vi "Main.vi"() -> ()   [LabVIEW 2015]
doc: "This template is for the Queued Message Handler design pattern.\n\nThe Event Handling Loop generates messages based on user interface actions.\n\nThe Message Handling Loop processes messages generated by the Event Handling Loop, or by other messages. The messages are string values, so new messages can be added easily to the Message Cases case structure in the Message Handling Loop. Each message cluster can also provide an optional value for Message Data, which is a variant that can be converted to whatever message-specific data is required."
uses:
  controls/UI Data.ctl
  support/Boiler System Globals.vi
  support/Message Queue/Message Queue.lvlib
  support/User Event - Stop/User Event - Stop.lvlib
  Boiler/Boiler.lvlib
panel:
  out "Display <Replace Me>":string
  in  "Do Something Else <Replace Me>":bool
  in  "Do Something <Replace Me>":bool
  in  "Stop Button":bool
  # "These controls have associated \"Value Changed\" events configured in the Event Structure on the diagram.\n\nReplace them (and reconfigure the Event Structure) with the controls you need for your application."
  # "This template is for the Queued Message Handler design pattern.\n\nSee the block diagram for more information on how to use this template."
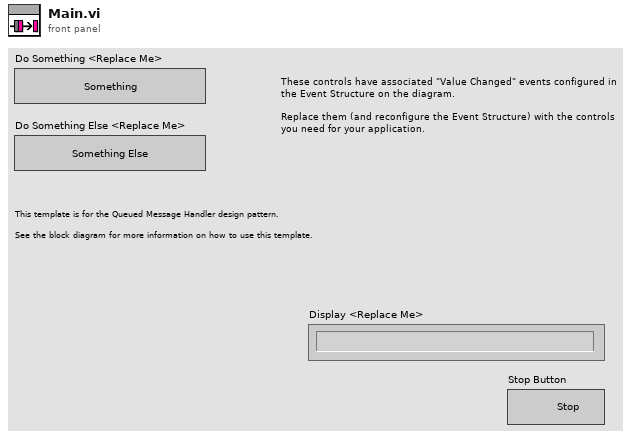
[diagram p1: front panel]
types:
  T1 = typedef "UI Data.ctl" = cluster{"Boolean <Replace Me>":bool, "String <Replace Me>":string, "Numeric <Replace Me>":dbl, "Do Something Ref":refnum<vi>, "Do Something Else Ref":refnum<vi>, "Data Display Ref":refnum<vi>, "Stop Button Ref":refnum<vi>}
  T2 = typedef "Notifiers.ctl" = cluster{"Handshake":refnum<notifier>, "Flame Level":refnum<notifier>, "Controller Exit":refnum<notifier>, "Boiler Exit":refnum<notifier>}
  T3 = typedef "Message Queue.lvlib/All Message Queues.ctl" = cluster{"MHL":refnum<queue>, "Boiler Controller":refnum<queue>, "Boiler":refnum<queue>}
  T4 = enum32{"invalid app kind", "Development System", "Run Time System", "Student Edition", "Embedded LabVIEW", "Evaluation", "Custom"}
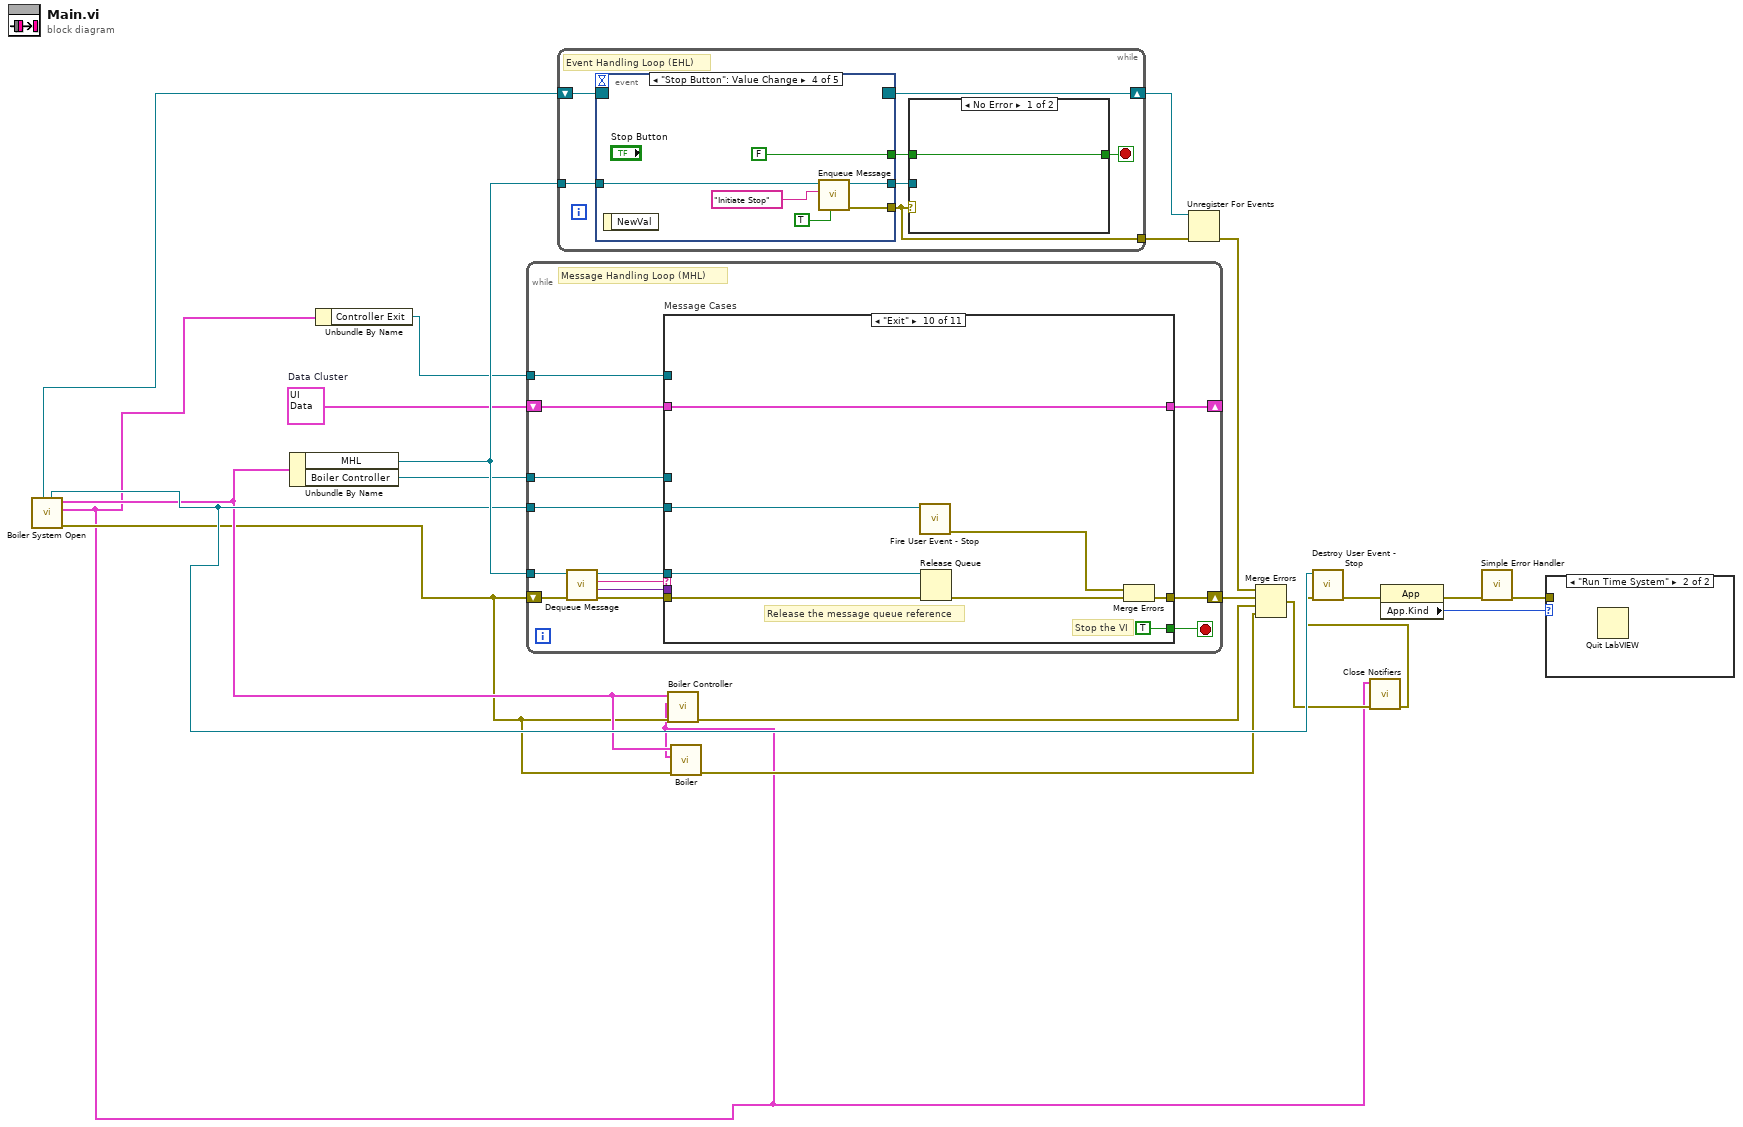
[diagram p0: block diagram]
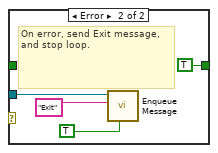
[diagram p3: hidden frame]
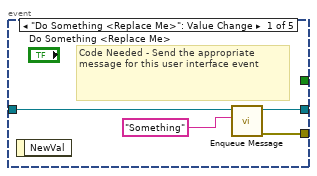
[diagram p4: hidden frame]
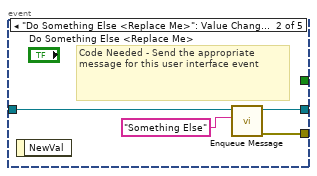
[diagram p5: hidden frame]
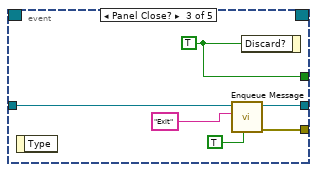
[diagram p6: hidden frame]
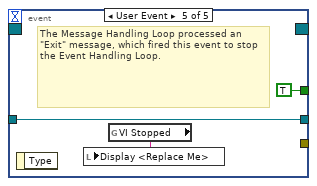
[diagram p7: hidden frame]
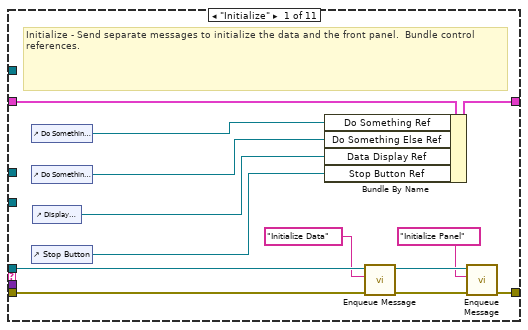
[diagram p8: hidden frame]
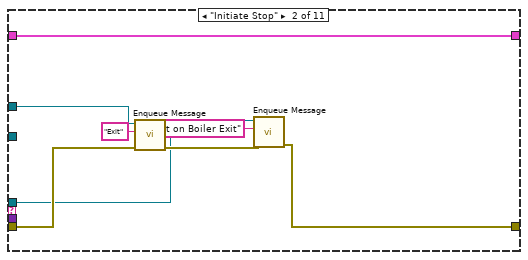
[diagram p9: hidden frame]
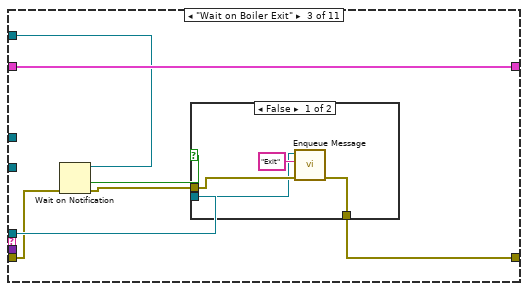
[diagram p10: hidden frame]
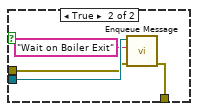
[diagram p11: hidden frame]
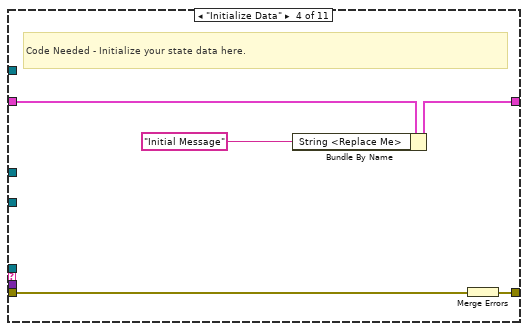
[diagram p12: hidden frame]
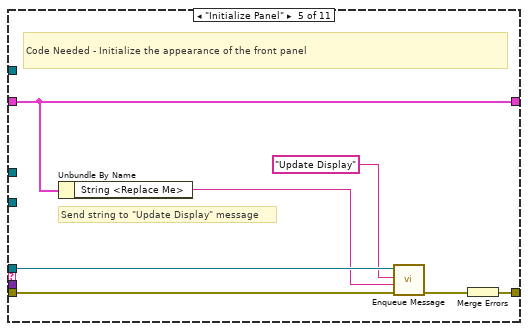
[diagram p13: hidden frame]
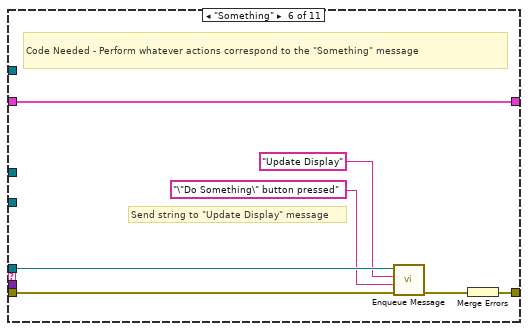
[diagram p14: hidden frame]
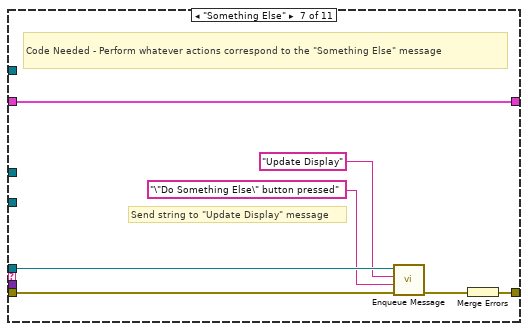
[diagram p15: hidden frame]
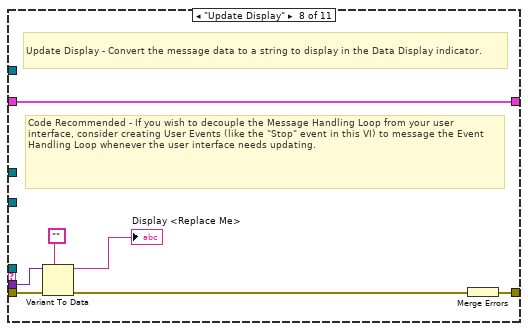
[diagram p16: hidden frame]
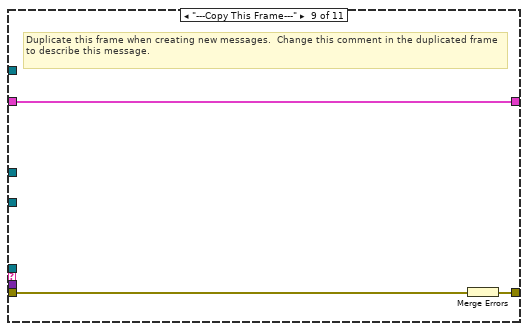
[diagram p17: hidden frame]
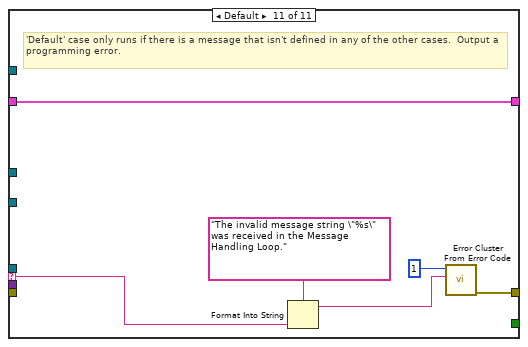
[diagram p18: hidden frame]
diagram:
  w15 = T1 {"Boolean <Replace Me>"=TRUE, "String <Replace Me>"="", "Numeric <Replace Me>"=0.0, "Do Something Ref"=refnum, "Do Something Else Ref"=refnum, "Data Display Ref"=refnum, "Stop Button Ref"=refnum}  # Data Cluster
  n1 = call "Boiler System Open.vi"() -> ("error out"=w6:errorcluster, "Notifiers"=w1:T2, "Message Queues"=w7:T3, "User Event - Stop"=w8:refnum<user-event>, "Stop Event Registration Refnum"=w9:refnum<event-registration>)  [unwired: 7 in]
  n2 = Unbundle By Name(w7) -> ("MHL"=w20:refnum<queue>, "Boiler Controller"=w13:refnum<queue>)
  n3 = Unbundle By Name(w1) -> ("Controller Exit"=w4:refnum<notifier>)
  n4 = while {
    tunnel: w20 -> [w24]
    shift-right: [w33] -> _
    shift-left: w15 -> [w34]
    tunnel: w8 -> [w30]
    shift-right: [w31] -> w21
    shift-left: w6 -> [w29]
    tunnel: w13 -> [w23]
    tunnel: w4 -> [w22]
    stop <- w32 stop-if-true
    # "Message Handling Loop (MHL)"
    n5 = call "Dequeue Message.vi"("error in (no error)"=w29, "Message Queue"=w24) -> ("error out"=w28:errorcluster, "Message Data"=w26:variant, "Message"=w27:string, "dup Message Queue"=w25:refnum<queue>)  [unwired: 6 in]
    n6 = case "Message Cases" shown="\"Exit\"" w27 {
      selector: w27 -> [_ _ _ _ _ _ _ _ _ _ w118]
      tunnel: w25 -> [w43 w49 w59 _ w79 w85 w92 _ _ w114 _]
      tunnel: w28 -> [w46 w51 w58 w75 w80 w87 w94 w101 w106 w107 _]
      tunnel: [w47 w50 w56 w71 w81 w88 w95 w102 w104 w110 w116] -> w31
      tunnel: w34 -> [w40 w55 w62 w74 w82 w89 w96 w103 w105 w113 w120]
      tunnel: [w39 w55 w62 w73 w82 w89 w96 w103 w105 w113 w120] -> w33
      tunnel: [_ _ _ _ _ _ _ _ _ TRUE _] -> w32
      tunnel: w26 -> [_ _ _ _ _ _ _ w100 _ _ _]
      tunnel: w30 -> [_ _ _ _ _ _ _ _ _ w109 _]
      tunnel: w23 -> [_ w54 _ _ _ _ _ _ _ _ _]
      tunnel: w22 -> [_ _ w61 _ _ _ _ _ _ _ _]
      frame "Initialize" {
        # "Initialize - Send separate messages to initialize the data and the front panel.  Bundle control references."
        n7 = control-ref of="Do Something <Replace Me>"() -> (w38:refnum<vi>)
        n8 = control-ref of="Do Something Else <Replace Me>"() -> (w37:refnum<vi>)
        n9 = control-ref of="Stop Button"() -> (w35:refnum<vi>)
        n10 = control-ref of="Display <Replace Me>"() -> (w36:refnum<vi>)
        n11 = Bundle By Name(cluster=w40, "Do Something Ref"=w38, "Do Something Else Ref"=w37, "Data Display Ref"=w36, "Stop Button Ref"=w35) -> (w39:T1)
        n12 = call "Enqueue Message.vi"("error in (no error)"=w46, "Message"="Initialize Data", "Message Queue"=w43) -> ("error out"=w45:errorcluster, "dup Message Queue"=w44:refnum<queue>)  [unwired: 7 in]
        n13 = call "Enqueue Message.vi"("error in (no error)"=w45, "Message"="Initialize Panel", "Message Queue"=w44) -> ("error out"=w47:errorcluster)  [unwired: 7 in, 1 out]
      }
      frame "Initiate Stop" {
        n14 = call "Enqueue Message.vi"("error in (no error)"=w51, "Message"="Exit", "Message Queue"=w54) -> ("error out"=w52:errorcluster)  [unwired: 7 in, 1 out]
        n15 = call "Enqueue Message.vi"("error in (no error)"=w52, "Message"="Wait on Boiler Exit", "Message Queue"=w49) -> ("error out"=w50:errorcluster)  [unwired: 7 in, 1 out]
      }
      frame "Wait on Boiler Exit" {
        n16 = Wait on Notification(notifier=w61, error in (no error)=w58) -> (timed out?=w60:bool, error out=w57:errorcluster)  [unwired: 2 in, 2 out]
        n17 = case shown="False" w60 {
          tunnel: w59 -> [w63 w70]
          tunnel: w57 -> [w65 w68]
          tunnel: [w64 w67] -> w56
          frame False {
            n18 = call "Enqueue Message.vi"("error in (no error)"=w65, "Message"="Exit", "Message Queue"=w63) -> ("error out"=w64:errorcluster)  [unwired: 7 in, 1 out]
          }
          frame True {
            n19 = call "Enqueue Message.vi"("error in (no error)"=w68, "Message"="Wait on Boiler Exit", "Message Queue"=w70) -> ("error out"=w67:errorcluster)  [unwired: 7 in, 1 out]
          }
        }
      }
      frame "Initialize Data" {
        # "Code Needed - Initialize your state data here."
        n20 = Bundle By Name(cluster=w74, "String <Replace Me>"="Initial Message" ("Initial Message")) -> (w73:T1)
        n21 = Merge Errors(w75) -> (w71:errorcluster)
      }
      frame "Initialize Panel" {
        # "Send string to \"Update Display\" message"
        # "Code Needed - Initialize the appearance of the front panel"
        n22 = Unbundle By Name(w82) -> ("String <Replace Me>"=w76:string)
        n23 = call "Enqueue Message.vi"("error in (no error)"=w80, "Message Data"=w76, "Message"="Update Display", "Message Queue"=w79) -> ("error out"=w78:errorcluster)  [unwired: 6 in, 1 out]
        n24 = Merge Errors(w78) -> (w81:errorcluster)
      }
      frame "Something" {
        # "Send string to \"Update Display\" message"
        # "Code Needed - Perform whatever actions correspond to the \"Something\" message"
        n25 = call "Enqueue Message.vi"("error in (no error)"=w87, "Message Data"="\"Do Something\" button pressed" ("\"Do Something\" button pressed"), "Message"="Update Display", "Message Queue"=w85) -> ("error out"=w86:errorcluster)  [unwired: 6 in, 1 out]
        n26 = Merge Errors(w86) -> (w88:errorcluster)
      }
      frame "Something Else" {
        # "Send string to \"Update Display\" message"
        # "Code Needed - Perform whatever actions correspond to the \"Something Else\" message"
        n27 = call "Enqueue Message.vi"("error in (no error)"=w94, "Message Data"="\"Do Something Else\" button pressed" ("\"Do Something Else\" button pressed"), "Message"="Update Display", "Message Queue"=w92) -> ("error out"=w93:errorcluster)  [unwired: 6 in, 1 out]
        n28 = Merge Errors(w93) -> (w95:errorcluster)
      }
      frame "Update Display" {
        # "Code Recommended - If you wish to decouple the Message Handling Loop from your user interface, consider creating User Events (like the \"Stop\" event in this VI) to message the Event Handling Loop whenever the user interface needs updating."
        # "Update Display - Convert the message data to a string to display in the Data Display indicator."
        n29 = Variant To Data(error in=w101, type="", Variant=w100) -> (data=→"Display <Replace Me>":string, error out=w98:errorcluster)
        n30 = Merge Errors(w98) -> (w102:errorcluster)
      }
      frame "---Copy This Frame---" {
        # "Duplicate this frame when creating new messages.  Change this comment in the duplicated frame to describe this message."
        n31 = Merge Errors(w106) -> (w104:errorcluster)
      }
      frame "Exit" {
        # "Stop the VI"
        # "Release the message queue reference"
        n32 = call "Fire User Event - Stop.vi"("User Event - Stop"=w109) -> ("error out"=w108:errorcluster)  [unwired: 10 in]
        n33 = Release Queue(queue=w114, error in (no error)=w107) -> (error out=w111:errorcluster)  [unwired: 1 in, 2 out]
        n34 = Merge Errors(w108, w111) -> (w110:errorcluster)
      }
      frame Default {
        # "'Default' case only runs if there is a message that isn't defined in any of the other cases.  Output a programming error."
        n35 = Format Into String(format string="The invalid message string \"%s\" was received in the Message Handling Loop." ("Unknown Message Error Text"), w118) -> (resulting string=w115:string)  [unwired: 2 in, 1 out]
        n36 = call <vilib>:"Error Cluster From Error Code.vi"("error message (\"\")"=w115, "error code (0)"=1) -> ("error out"=w116:errorcluster)  [unwired: 7 in]
      }
    }
  }
  n37 = while {
    tunnel: w20 -> [w127]
    tunnel: [w123] -> w17
    shift-right: [w121] -> w16
    shift-left: w9 -> [w122]
    stop <- w125 stop-if-true
    # "Event Handling Loop (EHL)"
    n38 = event shown="[3] \"Stop Button\": Value Change" {
      selector: w122 -> [_ _ _ _ _]
      dyn-events: [_ _ _ _ _] -> w121
      timeout: _ -> [_ _ _ _ _]
      tunnel: [_ _ w146 FALSE ("Discard?") TRUE ("Discard?")] -> w126
      tunnel: w127 -> [w136 w140 w145 w152 w155]
      tunnel: [w135 w138 w144 w151 _] -> w123
      tunnel: [w134 w139 w143 w149 w155] -> w124
      event "Do Something <Replace Me>": Value Change {
        # "Code Needed - Send the appropriate message for this user interface event"
        n39 = event-data() -> ()  [unwired: 1 in, 1 out]
        n40 = call "Enqueue Message.vi"("Message"="Something", "Message Queue"=w136) -> ("error out"=w135:errorcluster, "dup Message Queue"=w134:refnum<queue>)  [unwired: 8 in]
      }
      event "Do Something Else <Replace Me>": Value Change {
        # "Code Needed - Send the appropriate message for this user interface event"
        n41 = event-data() -> ()  [unwired: 1 in, 1 out]
        n42 = call "Enqueue Message.vi"("Message"="Something Else", "Message Queue"=w140) -> ("error out"=w138:errorcluster, "dup Message Queue"=w139:refnum<queue>)  [unwired: 8 in]
      }
      event Panel Close? {
        w146 = TRUE ("Discard?")
        n43 = event-data() -> ()  [unwired: 1 in, 1 out]
        n44 = call "Enqueue Message.vi"("Priority Message? (F)"=TRUE, "Message"="Exit", "Message Queue"=w145) -> ("error out"=w144:errorcluster, "dup Message Queue"=w143:refnum<queue>)  [unwired: 7 in]
        n45 = event-data("Discard?"=w146) -> ()  [unwired: 1 in, 1 out]
      }
      event "Stop Button": Value Change {
        n46 = event-data() -> ()  [unwired: 1 in, 1 out]
        n47 = call "Enqueue Message.vi"("Priority Message? (F)"=TRUE, "Message"="Initiate Stop", "Message Queue"=w152) -> ("error out"=w151:errorcluster, "dup Message Queue"=w149:refnum<queue>)  [unwired: 7 in]
      }
      event User Event {
        # "The Message Handling Loop processed an \"Exit\" message, which fired this event to stop the Event Handling Loop."
        n48 = event-data() -> ()  [unwired: 1 in, 1 out]
        n49 = global read "Boiler System Globals.vi" "VI Stopped"() -> (w153:string)
        n50 = local write "Display <Replace Me>"(w153) -> ()
      }
    }
    n51 = case shown="No Error" w123 {
      tunnel: [w128 TRUE ("Discard?")] -> w125
      tunnel: w126 -> [w128 _]
      tunnel: w124 -> [_ w131]
      frame No Error {
      }
      frame Error {
        # "On error, send Exit message, and stop loop."
        n52 = call "Enqueue Message.vi"("Priority Message? (F)"=TRUE, "Message"="Exit", "Message Queue"=w131) -> ()  [unwired: 7 in, 2 out]
      }
    }
  }
  n53 = call "Boiler Controller.vi"("error in"=w6, "Notifiers"=w1, "Message Queues"=w7) -> ("error out"=w14:errorcluster)  [unwired: 8 in]
  n54 = call "Boiler.vi"("error in"=w6, "Notifiers"=w1, "Message Queues"=w7) -> ("error out"=w5:errorcluster)  [unwired: 8 in]
  n55 = Unregister For Events(event registration refnum=w16, error in=w17) -> (error out=w18:errorcluster)
  n56 = Merge Errors(w18, w21, w14, w5) -> (w3:errorcluster)
  n57 = call "Close Notifiers.vi"("error in (no error)"=w3, "Cluster"=w1) -> ("error out"=w2:errorcluster)  [unwired: 9 in]
  n58 = call "Destroy User Event - Stop.vi"("error in (no error)"=w2, "User Event - Stop"=w8) -> ("error out"=w19:errorcluster)  [unwired: 9 in]
  n59 = property class="App"(error in=w19) -> (error out=w12:errorcluster, "App.Kind"=w11:T4)  [unwired: 1 in, 1 out]
  n60 = call <vilib>:"Simple Error Handler.vi"("error in (no error)"=w12) -> ("error out"=w10:errorcluster)  [unwired: 4 in, 4 out]
  n61 = case shown="\"Run Time System\"" w11 {
    tunnel: w10 -> [_ _]
    frame Default {
    }
    frame "Run Time System" {
      n62 = Quit LabVIEW() -> ()  [unwired: 1 in]
    }
  }
